vi "Determine Transition to Idle.vi"(0 "SV Signal in":refnum<class "SV Signal.lvclass">, 5 "samples generated at state in":u64, 7 "time offset at state in":dbl format="%#_13g", 11 "error in (no error)":errorcluster, 12 "signal state in":variant) -> (4 "SV Signal out":refnum<class "SV Signal.lvclass">, 6 "samples generated at state out":u64, 8 "time offset at state out":dbl format="%#_13g", 10 "generation state out":T1=enum."Pre-Measurement Settling", 13 "transitioned to Idle?":bool, 14 "signal state out":variant, 15 "error out":errorcluster)   [LabVIEW 2017, in "SV Signal.lvclass"]
uses:
  <vilib>/addons/_NISVFA/_Generation/Signal Generation/SV Signal/SV Signal.lvclass
  <vilib>/addons/_NISVFA/_Generation/Signal Generation/SV Signal/sv_Generation State.ctl
  <vilib>/addons/_NISVFA/_Generation/Signal Generation/SV Signal/SV Signal.lvclass/SV Signal.ctl
  <vilib>/addons/_NISVFA/_Generation/Signal Generation/SV Signal/sv_Signal State Attribute.ctl
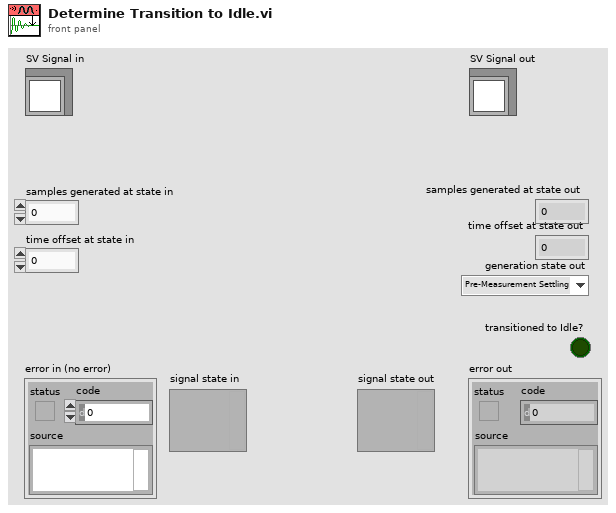
[diagram p1: front panel]
types:
  T1 = typedef "SV Signal.lvclass/sv_Generation State.ctl" = enum16{"Idle", "Ramp Up", "Pre-Measurement Settling", "Measurement", "Post-Measurement Settling", "Discrete Sweep Transition", "Ramp Down", "Update"}
  T2 = typedef "SV Signal.lvclass/sv_Signal State Attribute.ctl" = string
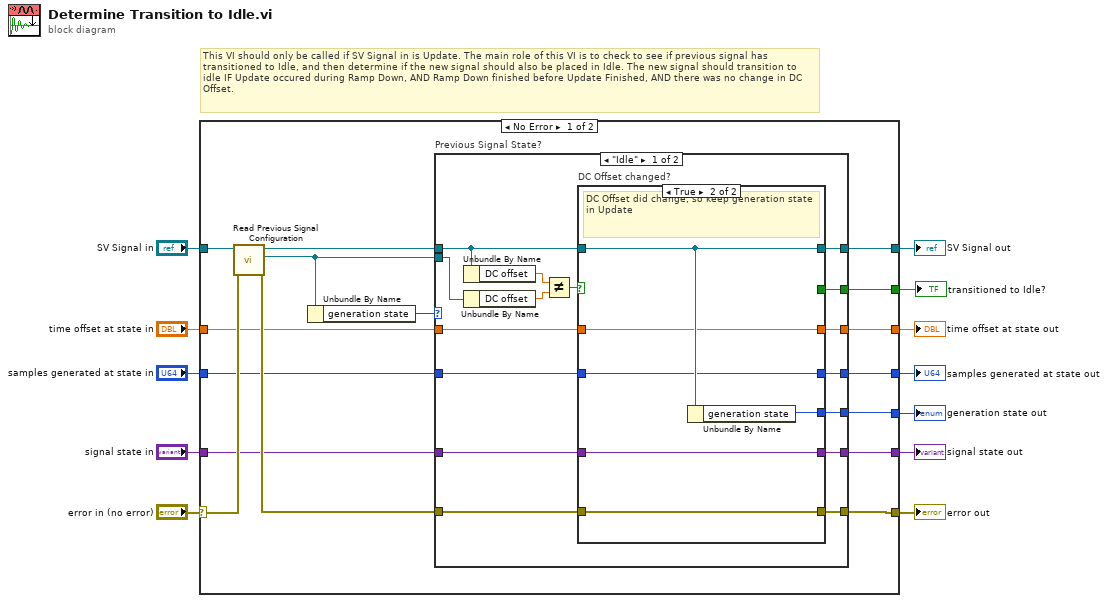
[diagram p0: block diagram]
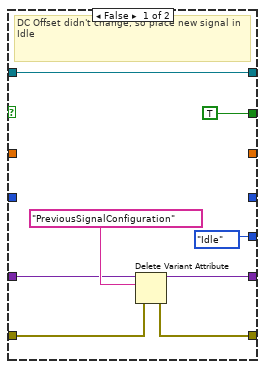
[diagram p2: hidden frame]
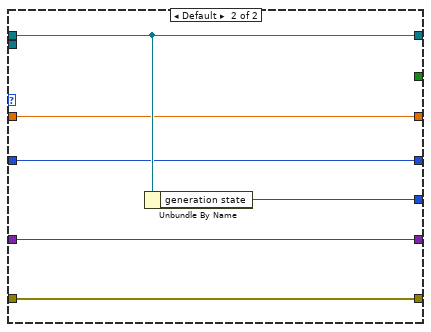
[diagram p3: hidden frame]
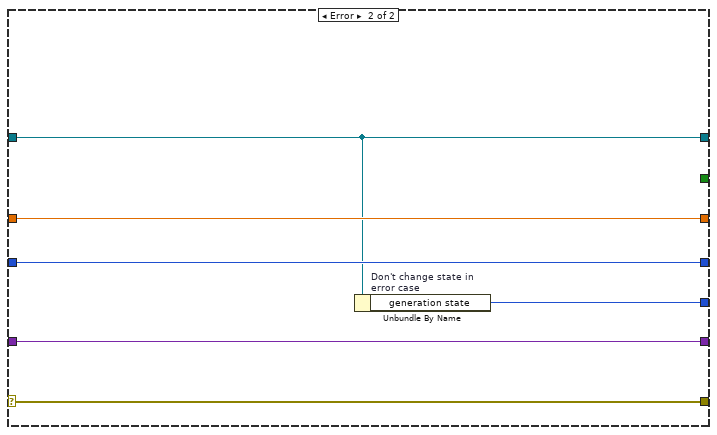
[diagram p4: hidden frame]
diagram:
  # "This VI should only be called if SV Signal in is Update. The main role of this VI is to check to see if previous signal has transitioned to Idle, and then determine if the new signal should also be placed in Idle. The new signal should transition to idle IF Update occured during Ramp Down, AND Ramp Down finished before Update Finished, AND there was no change in DC Offset."
  n1 = case shown="No Error" "error in (no error)" {
    selector: "error in (no error)" -> [w27 w70]
    tunnel: [w25 w70] -> w11
    tunnel: [w21 w66] -> w9
    tunnel: "SV Signal in" -> [w28 w66]
    tunnel: [w18 w69] -> w8
    tunnel: "time offset at state in" -> [w17 w69]
    tunnel: [w16 w68] -> w6
    tunnel: "samples generated at state in" -> [w15 w68]
    tunnel: "signal state in" -> [w22 w67]
    tunnel: [w23 w67] -> w3
    tunnel: [w19 w65] -> w2
    tunnel: [w13 _] -> w1
    frame No Error {
      n2 = call <vilib>:"Read Previous Signal Configuration.vi"("error in (no error)"=w27, "current signal configuration in"=w28) -> ("error out"=w24:errorcluster, "previous signal configuration"=w14:refnum<class "SV Signal.lvclass">, "current signal configuration out"=w20:refnum<class "SV Signal.lvclass">)  [unwired: 7 in]
      n3 = Unbundle By Name(w14) -> ("generation state"=w26:T1)
      n4 = case "Previous Signal State?" shown="\"Idle\"" w26 {
        tunnel: [w31 w64] -> w25
        tunnel: w24 -> [w30 w64]
        tunnel: [w33 w63] -> w23
        tunnel: w22 -> [w32 w63]
        tunnel: [w40 w62] -> w21
        tunnel: w20 -> [w39 w62]
        tunnel: [w38 w61] -> w19
        tunnel: [w37 w60] -> w18
        tunnel: w17 -> [w36 w60]
        tunnel: [w35 w59] -> w16
        tunnel: w15 -> [w34 w59]
        tunnel: w14 -> [w44 _]
        tunnel: [w29 _] -> w13
        frame "Idle" {
          n5 = Unbundle By Name(w39) -> ("DC offset"=w43:dbl)
          n6 = Unbundle By Name(w44) -> ("DC offset"=w42:dbl)
          n7 = Not Equal?(x=w43, y=w42) -> (x != y?=w41:bool)
          n8 = case "DC Offset changed?" shown="True" w41 {
            tunnel: [w52 w58] -> w40
            tunnel: w39 -> [w52 w58]
            tunnel: [sv_Generation_State."Idle" ("generation state") w57] -> w38
            tunnel: [_ w56] -> w37
            tunnel: w36 -> [_ w56]
            tunnel: [_ w55] -> w35
            tunnel: w34 -> [_ w55]
            tunnel: [w46 w54] -> w33
            tunnel: w32 -> [w49 w54]
            tunnel: [w47 w53] -> w31
            tunnel: w30 -> [w48 w53]
            tunnel: [TRUE _] -> w29
            frame False {
              # "DC Offset didn't change, so place new signal in Idle"
              n9 = Delete Variant Attribute(4:w48, 6:T2 "PreviousSignalConfiguration" ("name (all attributes)"), 7:w49) -> (0:w47:errorcluster, 3:w46:variant)  [unwired: 1 out]
            }
            frame True {
              # "DC Offset did change, so keep generation state in Update"
              n10 = Unbundle By Name(w58) -> ("generation state"=w57:T1)
            }
          }
        }
        frame Default {
          n11 = Unbundle By Name(w62) -> ("generation state"=w61:T1)
        }
      }
    }
    frame Error {
      n12 = Unbundle By Name "Don't change state in error case"(w66) -> ("generation state"=w65:T1)
    }
  }
  "error out" <- w11
  "SV Signal out" <- w9
  "time offset at state out" <- w8
  "samples generated at state out" <- w6
  "generation state out" <- w2
  "signal state out" <- w3
  "transitioned to Idle?" <- w1
